vi "factorial (разные способы).vi"() -> ()   [LabVIEW 2017]
uses:
  <vilib>/imath/engines/lvmath2/RunTimeEngine/NodeEndStatement/NIMS_NodeEndStatement_Output.vi
  <instcachedir>/0/NIMS_NodeEndStatement_Output_53EC0D466D134D7ABD903AC30B43404B.lvgen/NIMS_NodeEndStatement_Output_53EC0D466D134D7ABD903AC30B43404B_001.vi
  <vilib>/imath/engines/lvmath2/RunTimeEngine/ErrorHandling/NIMS_Finalize Error.vi
  fact.dll
  <vilib>/gmath/NI_Gmath.lvlib
panel:
  out "N ! (Подпрограмма \"штатная\")":dbl format="%^_8g"
  out "N! (Mathscript)":u64
  out "n!(Feedback)":i32
  out "N ! (Подпрограмма LV, SubVI)":u64
  in  "Предупреждать":bool
  out "N! (DLLl)":u64
  out "N! (формула)":u64
  out "N! (табулирование)":u64
  out "n! (массив)":u64
  out "n! (лок. пер)":u64
  out "n! (регистры сдвига)":dbl format="%^_8g"
  in  "N":i32
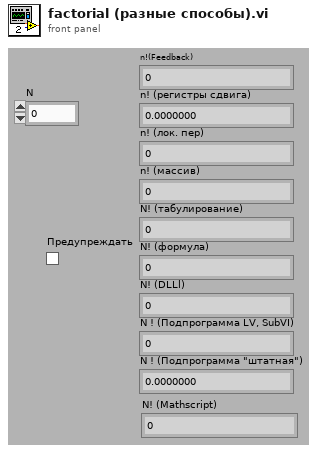
[diagram p1: front panel]
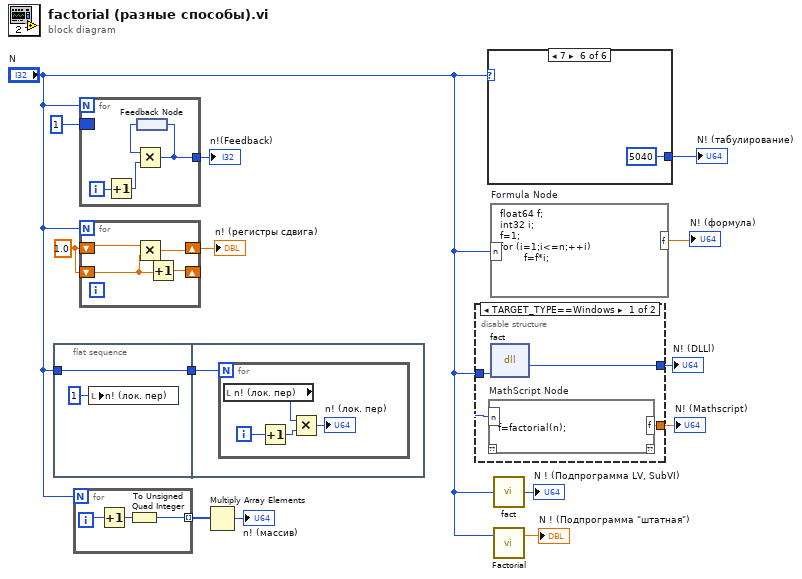
[diagram p0: block diagram]
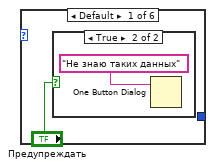
[diagram p3: hidden frame]
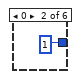
[diagram p5: hidden frame]
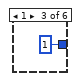
[diagram p6: hidden frame]
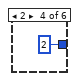
[diagram p7: hidden frame]
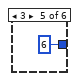
[diagram p8: hidden frame]
diagram:
  w1 = 1.0
  n1 = flat-sequence {
    tunnel: "N" -> [w16]
    tunnel: [w16] -> w4
    tunnel: w4 -> [w17]
    frame #0 {
      n2 = local write "n! (лок. пер)"(u64 1 ("n! (лок. пер)")) -> ()
    }
    frame #1 {
      n3 = for {
        N: w17 -> [_]
        i -> [w21]
        n4 = local read "n! (лок. пер)"() -> (w20:u64)
        n5 = Increment(x=w21) -> (x+1=w19:i32)
        n6 = Multiply(x=w20, y=w19) -> (x*y=→"n! (лок. пер)":u64)
      }
    }
  }
  n7 = for {
    N: "N" -> [_]
    tunnel: [w22] -> w13 mode=indexing
    i -> [w24]
    n8 = Increment(x=w24) -> (x+1=w23:i32)
    n9 = To Unsigned Quad Integer(1:w23) -> (0:w22:u64)
  }
  n10 = for {
    N: "N" -> [_]
    tunnel: [w25] -> w7
    border: 1 -> [_]
    i -> [w28]
    n11 = Increment(x=w28) -> (x+1=w27:i32)
    n12 = feedback #1() -> (w26:i32)
    n13 = Multiply(x=w26, y=w27) -> (x*y=w25:i32)
    n14 = feedback-in #1(w25) -> ()
  }
  "n!(Feedback)" <- w7
  n15 = for {
    N: "N" -> [_]
    shift-right: [w31] -> w14
    shift-left: w1 -> [w32]
    shift-right: [w30] -> _
    shift-left: w1 -> [w29]
    n16 = Multiply(x=w32, y=w29) -> (x*y=w31:dbl)
    n17 = Increment(x=w29) -> (x+1=w30:dbl)
  }
  "n! (регистры сдвига)" <- w14
  n18 = Multiply Array Elements(1:w13) -> (0:→"n! (массив)":u64)
  n19 = disable-structure shown="TARGET_TYPE==Windows" {
    disable-tunnel: [w35 _] -> w9
    disable-tunnel: "N" -> [w34 _]
    disable-tunnel: [w33 _] -> w2
    frame condition #0 (active) {
      n20 = mathscript code="f=factorial(n);"("n"=w34) -> ("f"=w33:dbl)  [unwired: 2 out]
      n21 = dll-call lib="PTH2Wabs D_iDriveDriveYandexЗагрузкиColledgeФакториалfact.dll" fn="fact" label="long fact(long n);"("n"=w34) -> (w35:i32)  [unwired: 4 in, 2 out]
    }
    frame condition #1 {
    }
  }
  "N! (DLLl)" <- w9
  "N! (Mathscript)" <- w2
  n22 = case shown="7" "N" {
    tunnel: [_ 1 1 2 6 5040] -> w11
    frame Default {
      n23 = case shown="True" "Предупреждать" {
        frame False {
        }
        frame True {
          n24 = One Button Dialog(message="Не знаю таких данных") -> ()  [unwired: 2 out]
        }
      }
    }
    frame 0 {
    }
    frame 1 {
    }
    frame 2 {
    }
    frame 3 {
    }
    frame 7 {
    }
  }
  "N! (табулирование)" <- w11
  n25 = formula code="float64 f;\nint32 i;\nf=1;\nfor (i=1;i<=n;++i)    \n        f=f*i;"("n"="N") -> ("f"=→"N! (формула)":dbl)
  n26 = call "fact.vi"("N"="N") -> ("N !"=→"N ! (Подпрограмма LV, SubVI)":u64)
  n27 = call <vilib>:"Factorial.vi"("n"="N") -> ("n!"=→"N ! (Подпрограмма \"штатная\")":dbl)  [unwired: 2 out]
